vi "大富翁.vi"() -> ()   [LabVIEW 2014]
panel:
  out "白色恐怖?":bool
  out "換誰?":dbl=1.0
  out "按鈕?":dbl
  in  "離開遊戲":bool
  out "骰子":dbl=6.0
  in  "遊戲人數":dbl=4.0
  out "位置 4":dbl
  out "剩幾天 4":dbl
  in  "入獄 4":bool=TRUE
  in  "擲骰子 4":bool
  out "位置 3":dbl
  out "剩幾天 3":dbl
  in  "入獄 3":bool=TRUE
  in  "擲骰子 3":bool
  out "位置 2":dbl
  out "剩幾天 2":dbl
  in  "入獄 2":bool=TRUE
  in  "擲骰子 2":bool
  out "P2指示":bool=TRUE
  out "玩家二財產":dbl
  out "位置 1":dbl
  in  "入獄 1":bool=TRUE
  out "剩幾天 1":dbl
  in  "擲骰子 1":bool=TRUE
  out "P4 棋子":bool=TRUE
  out "P3 棋子":bool=TRUE
  out "P2 棋子":bool=TRUE
  out "P1 棋子":bool
  out "P4指示":bool=TRUE
  out "玩家四財產":dbl
  out "P3指示":bool=TRUE
  out "玩家三財產":dbl
  out "P1指示":bool
  out "玩家一財產":dbl
  in  "中壢市":bool
  in  "新竹市":bool
  in  "新竹縣":bool
  in  "苗栗縣":bool
  in  "台中市":bool
  in  "南投縣":bool
  in  "彰化縣":bool
  in  "雲林縣":bool
  in  "嘉義市":bool
  in  "澎湖縣":bool
  in  "嘉義縣":bool
  in  "阿里山":bool
  in  "台南市":bool
  in  "高雄市":bool
  out "高雄市所有":u32(colorbox)=16777215
  out "中壢市所有":u32(colorbox)=16777215
  out "新竹市所有":u32(colorbox)=16777215
  out "新竹縣所有":u32(colorbox)=16777215
  out "苗栗縣所有":u32(colorbox)=16777215
  out "台中市所有":u32(colorbox)=16777215
  out "南投縣所有":u32(colorbox)=16777215
  out "彰化縣所有":u32(colorbox)=16777215
  out "雲林縣所有":u32(colorbox)=16777215
  out "嘉義市所有":u32(colorbox)=16777215
  out "澎湖縣所有":u32(colorbox)=16777215
  out "嘉義縣所有":u32(colorbox)=16777215
  out "阿里山所有":u32(colorbox)=16777215
  out "台南市所有":u32(colorbox)=16777215
  in  "屏東縣":bool
  out "屏東縣所有":u32(colorbox)=16777215
  in  "¾Á¤B":bool
  out "墾丁所有":u32(colorbox)=16777215
  in  "小琉球":bool
  in  "馬祖":bool
  in  "金門":bool
  in  "蘭嶼":bool
  in  "綠島":bool
  in  "台東縣":bool
  in  "花蓮縣":bool
  in  "宜蘭縣":bool
  in  "基隆市":bool
  in  "台北市":bool
  in  "新北市":bool
  in  "桃園市":bool
  out "桃園市所有":u32(colorbox)=16777215
  out "17旅4":bool
  out "17旅3":bool
  out "17旅2":bool
  out "17旅1":bool
  out "17房4":bool
  out "17房3":bool
  out "17房2":bool
  out "17房1":bool
  out "17¾Á¤B":u32(colorbox)=16777215
  out "19公園":u32(colorbox)=4417863
  out "32入獄":u32(colorbox)=6710886
  out "13監獄":u32(colorbox)=13553358
  out "28命運":u32(colorbox)=12155079
  out "18旅4":bool
  out "18旅3":bool
  out "18旅2":bool
  out "18旅1":bool
  out "18房4":bool
  out "18房3":bool
  out "18房2":bool
  out "18房1":bool
  out "18屏東縣":u32(colorbox)=16777215
  out "16命運":u32(colorbox)=12155079
  out "15旅4":bool
  out "15旅3":bool
  out "15旅2":bool
  out "15旅1":bool
  out "15房4":bool
  out "15房3":bool
  out "15房2":bool
  out "15房1":bool
  out "15小琉球":u32(colorbox)=16777215
  out "35機會":u32(colorbox)=51382
  out "14旅4":bool
  out "14旅3":bool
  out "14旅2":bool
  out "14旅1":bool
  out "14房4":bool
  out "14房3":bool
  out "14房2":bool
  out "14房1":bool
  out "33旅4":bool
  out "33旅3":bool
  out "33旅2":bool
  out "33旅1":bool
  out "33房4":bool
  out "33房3":bool
  out "33房2":bool
  out "33房1":bool
  out "33苗栗縣":u32(colorbox)=16776096
  out "34旅4":bool
  out "34旅3":bool
  out "34旅2":bool
  out "34旅1":bool
  out "34房4":bool
  out "34房3":bool
  out "34房2":bool
  out "34房1":bool
  out "34新竹縣":u32(colorbox)=4377855
  out "36旅4":bool
  out "36旅3":bool
  out "36旅2":bool
  out "36旅1":bool
  out "36房4":bool
  out "36房3":bool
  out "36房2":bool
  out "36房1":bool
  out "36新竹市":u32(colorbox)=10551209
  out "37旅4":bool
  out "37旅3":bool
  out "37旅2":bool
  out "37旅1":bool
  out "37房4":bool
  out "37房3":bool
  out "37房2":bool
  out "37房1":bool
  out "37中壢市":u32(colorbox)=16740729
  out "0起點":u32(colorbox)=16740906
  out "20旅4":bool
  out "20旅3":bool
  out "20旅2":bool
  out "20旅1":bool
  out "20房4":bool
  out "20房3":bool
  out "20房2":bool
  out "20房1":bool
  out "20高雄市":u32(colorbox)=16777215
  out "21旅4":bool
  out "21旅3":bool
  out "21旅2":bool
  out "21旅1":bool
  out "21房4":bool
  out "21房3":bool
  out "21房2":bool
  out "21房1":bool
  out "21台南市":u32(colorbox)=16777215
  out "12旅4":bool
  out "12旅3":bool
  out "12旅2":bool
  out "12旅1":bool
  out "12房4":bool
  out "12房3":bool
  out "12房2":bool
  out "12房1":bool
  out "12金門":u32(colorbox)=16777215
  out "11旅4":bool
  out "11旅3":bool
  out "11旅2":bool
  out "11旅1":bool
  out "11房4":bool
  out "11房3":bool
  out "11房2":bool
  out "11房1":bool
  out "11蘭嶼":u32(colorbox)=16777215
  out "10旅4":bool
  out "10旅3":bool
  out "10旅2":bool
  out "10旅1":bool
  out "10房4":bool
  out "10房3":bool
  out "10房2":bool
  out "10房1":bool
  out "10綠島":u32(colorbox)=16777215
  out "9旅4":bool
  out "9旅3":bool
  out "9旅2":bool
  out "9旅1":bool
  out "9房4":bool
  out "9房3":bool
  out "9房2":bool
  out "9房1":bool
  out "9台東縣":u32(colorbox)=16777215
  out "7旅4":bool
  out "7旅3":bool
  out "7旅2":bool
  out "7旅1":bool
  out "7房4":bool
  out "7房3":bool
  out "7房2":bool
  out "7房1":bool
  out "7花蓮縣":u32(colorbox)=16777215
  out "8機會":u32(colorbox)=51382
  out "5命運":u32(colorbox)=12155079
  out "6旅4":bool
  out "6旅3":bool
  out "6旅2":bool
  out "6旅1":bool
  out "6房4":bool
  out "6房3":bool
  out "6房2":bool
  out "6房1":bool
  out "6宜蘭縣":u32(colorbox)=16777215
  out "4旅4":bool
  out "4旅3":bool
  out "4旅2":bool
  out "4旅1":bool
  out "4房4":bool
  out "4房3":bool
  out "4房2":bool
  out "4房1":bool
  out "4基隆市":u32(colorbox)=16777215
  out "3旅4":bool
  out "3旅3":bool
  out "3旅2":bool
  out "3旅1":bool
  out "3房4":bool
  out "3房3":bool
  out "3房2":bool
  out "3房1":bool
  out "3台北市":u32(colorbox)=16777215
  out "2旅4":bool
  out "2旅3":bool
  out "2旅2":bool
  out "2旅1":bool
  out "2房4":bool
  out "2房3":bool
  out "2房2":bool
  out "2房1":bool
  out "2新北市":u32(colorbox)=16777215
  out "1旅4":bool
  out "1旅3":bool
  out "1旅2":bool
  out "1旅1":bool
  out "1房4":bool
  out "1房3":bool
  out "1房2":bool
  out "1房1":bool
  out "1桃園市":u32(colorbox)=16777215
  out "24機會":u32(colorbox)=51382
  out "22旅4":bool
  out "22旅3":bool
  out "22旅2":bool
  out "22旅1":bool
  out "22房4":bool
  out "22房3":bool
  out "22房2":bool
  out "22房1":bool
  out "22阿里山":u32(colorbox)=16777215
  out "23旅4":bool
  out "23旅3":bool
  out "23旅2":bool
  out "23旅1":bool
  out "23房4":bool
  out "23房3":bool
  out "23房2":bool
  out "23房1":bool
  out "23嘉義縣":u32(colorbox)=16777215
  out "25旅4":bool
  out "25旅3":bool
  out "25旅2":bool
  out "25旅1":bool
  out "25房4":bool
  out "25房3":bool
  out "25房2":bool
  out "25房1":bool
  out "25澎湖縣":u32(colorbox)=16777215
  out "26旅4":bool
  out "26旅3":bool
  out "26旅2":bool
  out "26旅1":bool
  out "26房4":bool
  out "26房3":bool
  out "26房2":bool
  out "26房1":bool
  out "26嘉義市":u32(colorbox)=16777215
  out "27旅4":bool
  out "27旅3":bool
  out "27旅2":bool
  out "27旅1":bool
  out "27房4":bool
  out "27房3":bool
  out "27房2":bool
  out "27房1":bool
  out "29旅4":bool
  out "29旅3":bool
  out "29旅2":bool
  out "29旅1":bool
  out "29房4":bool
  out "29房3":bool
  out "29房2":bool
  out "29房1":bool
  out "29彰化縣":u32(colorbox)=16777215
  out "30旅4":bool
  out "30旅3":bool
  out "30旅2":bool
  out "30旅1":bool
  out "30房4":bool
  out "30房3":bool
  out "30房2":bool
  out "30房1":bool
  out "31旅4":bool
  out "31旅3":bool
  out "31旅2":bool
  out "31旅1":bool
  out "31房4":bool
  out "31房3":bool
  out "31房2":bool
  out "31房1":bool
  out "31台中市":u32(colorbox)=16777215
  out "新北市所有":u32(colorbox)=16777215
  out "小琉球所有":u32(colorbox)=16777215
  out "馬祖所有":u32(colorbox)=16777215
  out "金門縣所有":u32(colorbox)=16777215
  out "蘭嶼所有":u32(colorbox)=16777215
  out "綠島所有":u32(colorbox)=16777215
  out "台東縣所有":u32(colorbox)=16777215
  out "花蓮縣所有":u32(colorbox)=16777215
  out "宜蘭縣所有":u32(colorbox)=16777215
  out "基隆市所有":u32(colorbox)=16777215
  out "台北市所有":u32(colorbox)=16777215
  out "14馬祖":u32(colorbox)=16777215
  out "30南投縣":u32(colorbox)=16777215
  out "27雲林縣":u32(colorbox)=16777215
  out "背景":u32(colorbox)=11121611
  # "起點"
  # "桃園市"
  # "新北市"
  # "台北市"
  # "基隆市"
  # "命運"
  # "宜蘭縣"
  # "花蓮縣"
  # "機會"
  # "台東縣"
  # "綠島"
  # "蘭嶼"
  # "金門"
  # "$1000"
  # "$1500"
  # "$2000"
  # "$750"
  # "$800"
  # "$700"
  # "$650"
  # "$1100"
  # "$800"
  # "$600"
  # "通過+2000!!"
  # "¤¤\nÃc\n¥«"
  # "馬\n祖"
  # "$1000"
  # "$600"
  # "新\n竹\n市"
  # "¤p\n¯[\n²y"
  # "$1300"
  # "$900"
  # "機\n會"
  # "命\n運"
  # "新\n竹\n縣"
  # "¾Á\n¤B"
  # "$900"
  # "$900"
  # "屏\n東\n縣"
  # "­]\n®ß\n¿¤"
  # "$650"
  # "$800"
  # "$1200"
  # "$700"
  # "$750"
  # "$650"
  # "$850"
  # "$900"
  # "$700"
  # "$800"
  # "$1000"
  # "$1800"
  # "台中市"
  # "彰化縣"
  # "嘉義市"
  # "澎湖縣"
  # "機會"
  # "嘉義縣"
  # "阿里山"
  # "台南市"
  # "高雄市"
  # "公園"
  # "入獄"
  # "監獄"
  # "命運"
  # "南投縣"
  # "雲林縣"
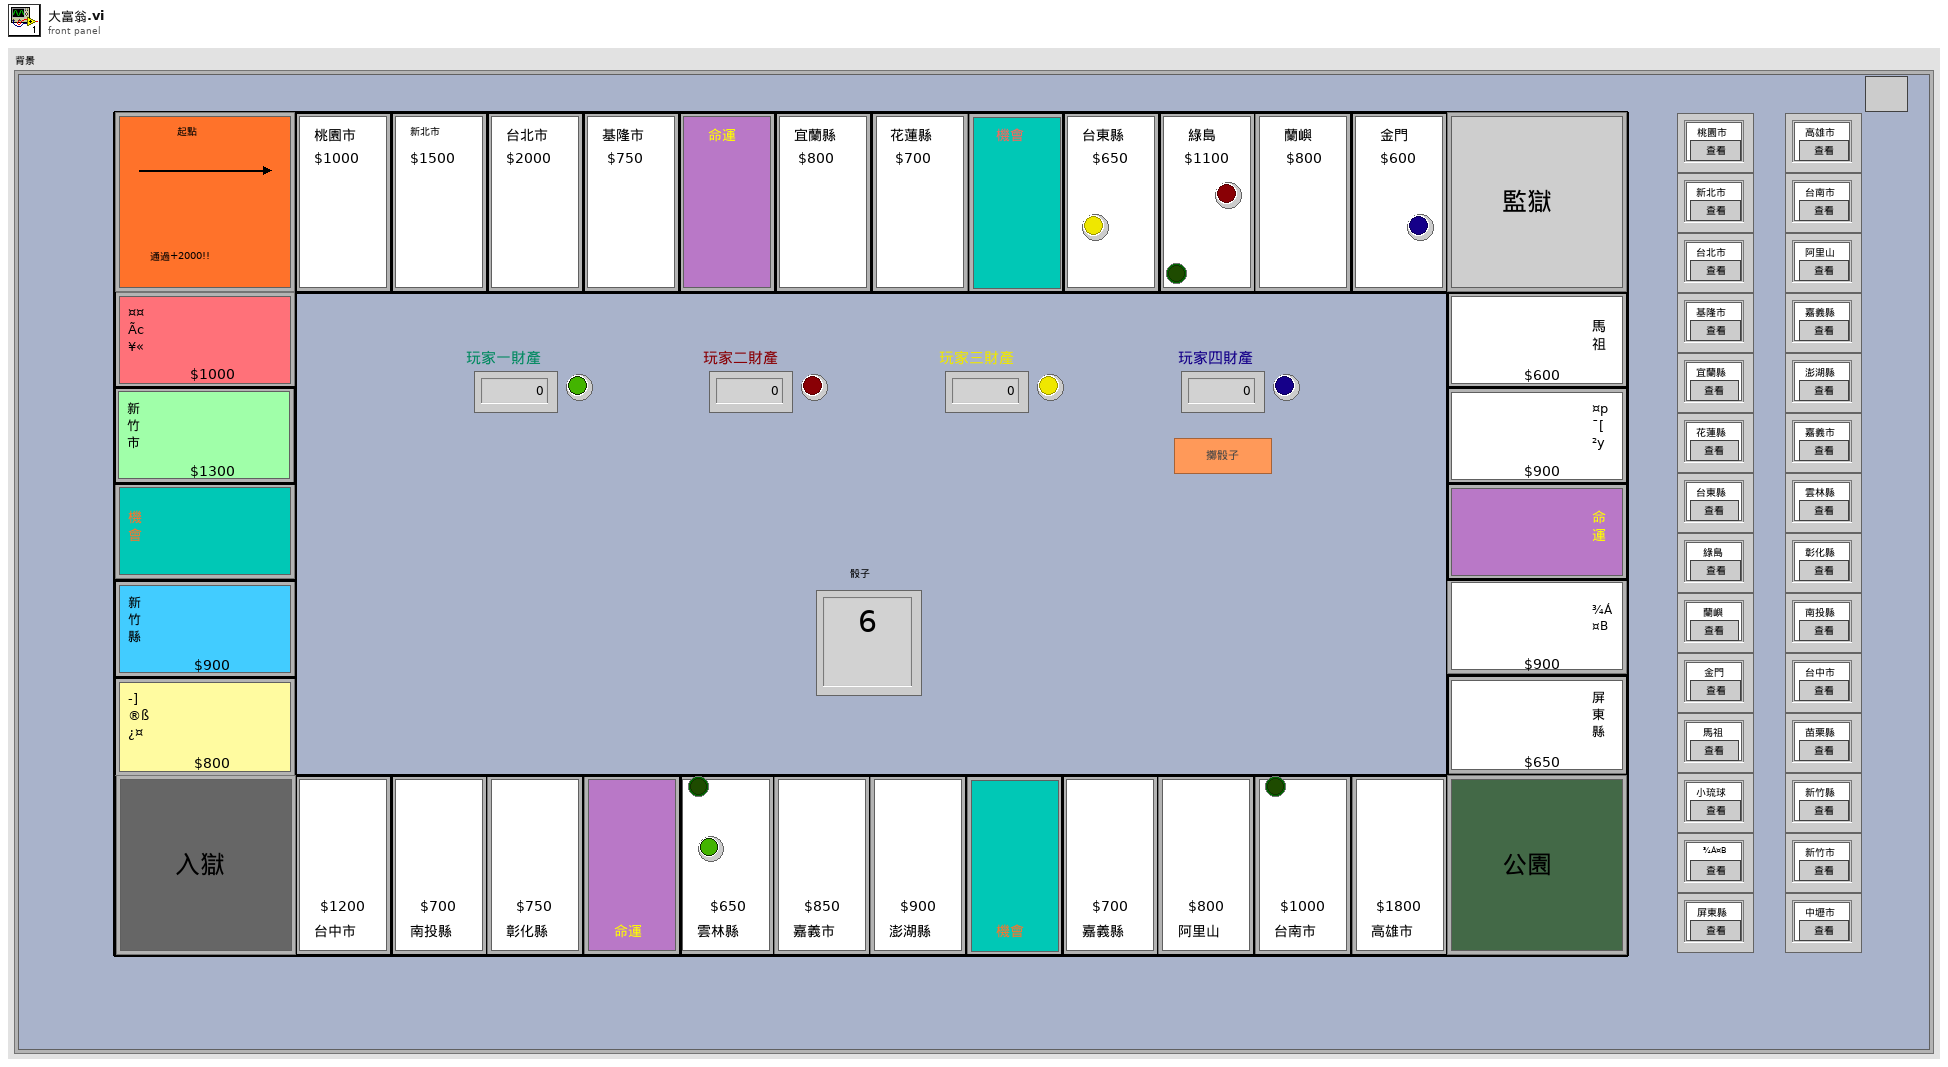
[diagram p1: front panel]
types:
  T1 = enum8{"Enabled", "Disabled", "Disabled and Grayed Out"}
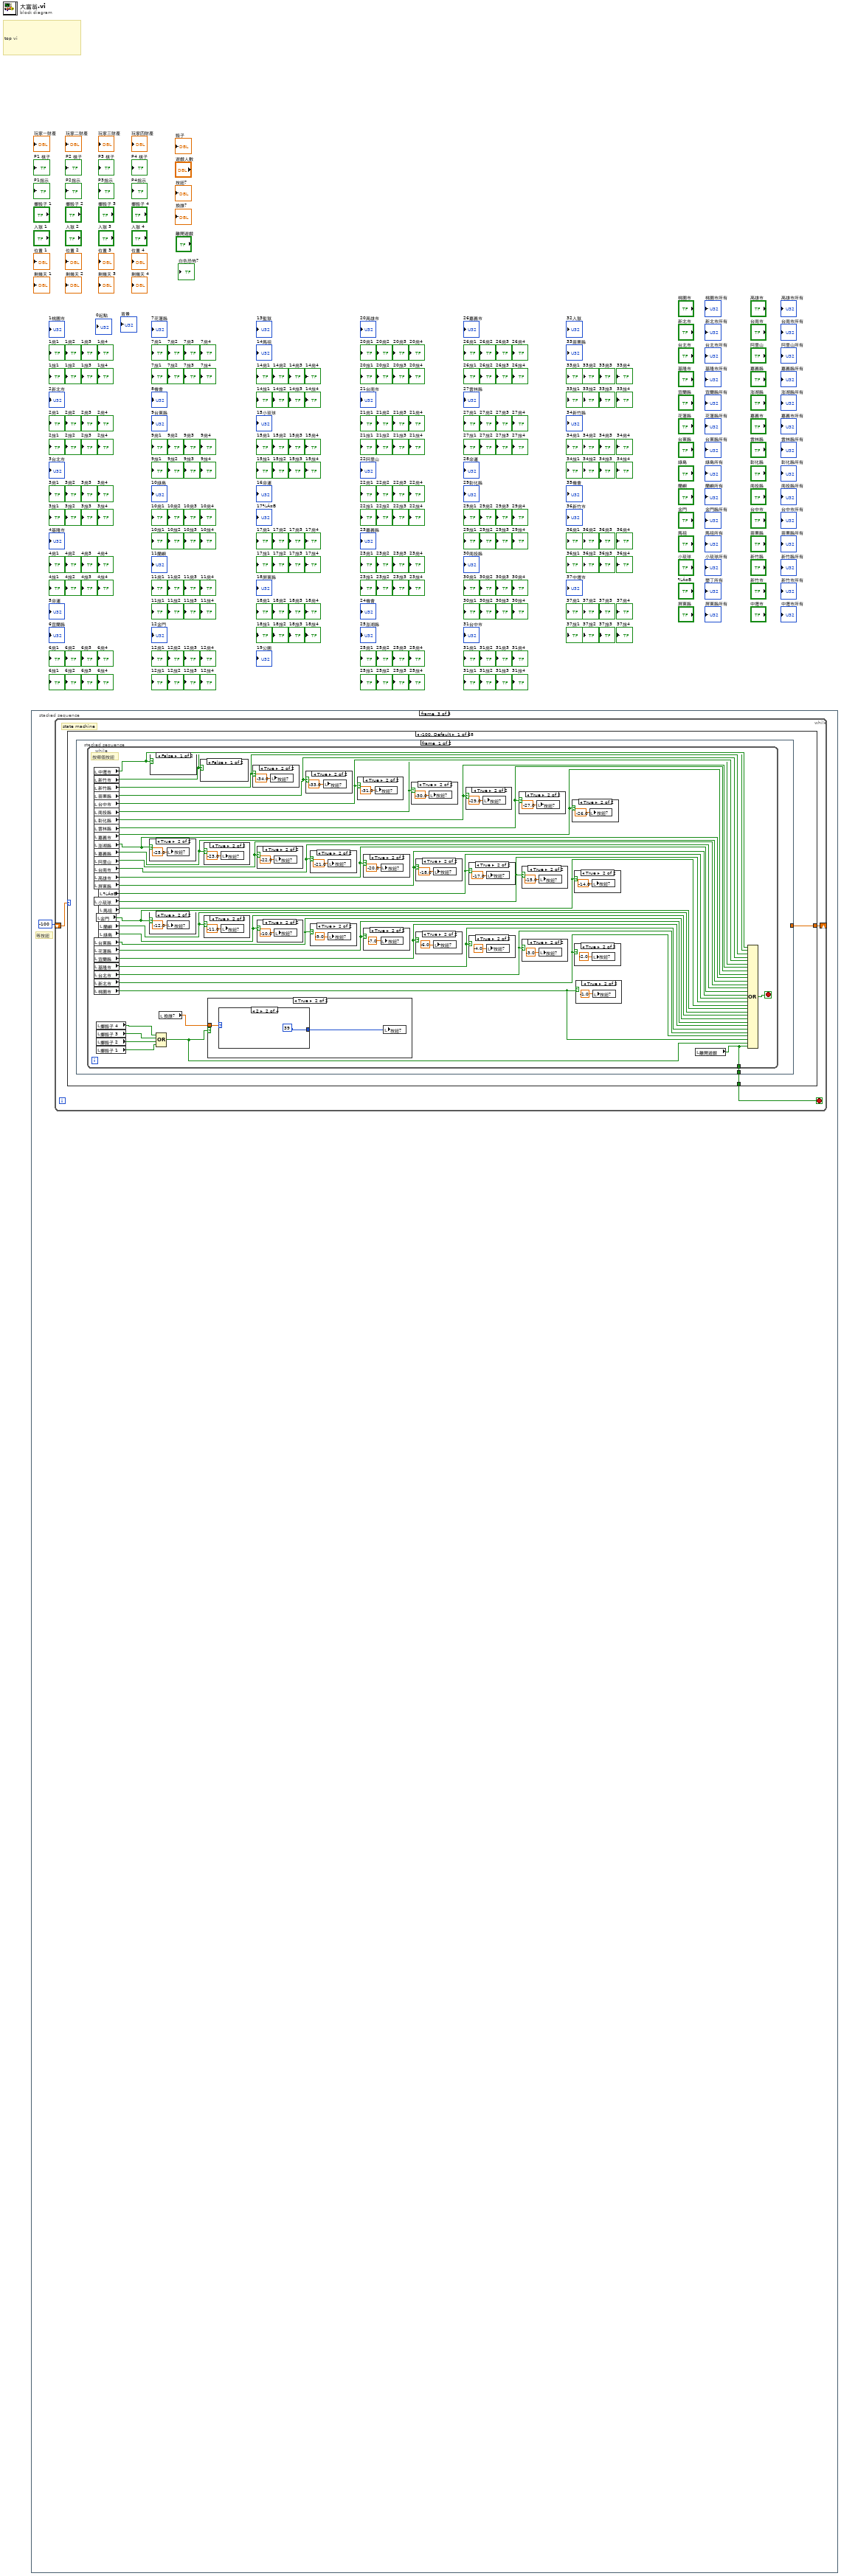
[diagram p0: block diagram]
diagram:
  # "top vi"
  n1 = stacked-sequence {
    frame #0 {
      w3 = TRUE ("P4 棋子")
      w5 = 144 ("Position:Top")
      w6 = 197 ("Position:Left")
      w7 = 112 ("Position:Top")
      w4 = 160 ("Position:Left")
      w8 = 15000.0 ("玩家四財產")
      w9 = FALSE
      w10 = 0.0 ("位置 4")
      w13 = u32 12155079 ("28命運")
      w12 = FALSE ("擲骰子 4")
      w14 = TRUE
      w15 = FALSE
      w17 = FALSE ("Visible")
      w18 = FALSE ("Visible")
      w19 = FALSE ("Visible")
      w20 = FALSE ("Visible")
      w22 = FALSE ("中壢市")
      w21 = FALSE ("Visible")
      w23 = FALSE ("Visible")
      w24 = FALSE
      w25 = u32 16777215 ("中壢市所有")
      w31 = u32 51382 ("地機會")
      w16 = FALSE
      n2 = local write "31旅4"(w16) -> ()
      n3 = local write "31旅3"(w16) -> ()
      n4 = local write "31旅2"(w16) -> ()
      n5 = local write "31旅1"(w16) -> ()
      n6 = local write "31房4"(w16) -> ()
      n7 = local write "31房3"(w16) -> ()
      n8 = local write "31房2"(w16) -> ()
      n9 = local write "31房1"(w16) -> ()
      n10 = local write "30旅4"(w16) -> ()
      n11 = local write "30旅3"(w16) -> ()
      n12 = local write "30旅2"(w16) -> ()
      n13 = local write "30旅1"(w16) -> ()
      n14 = local write "30房4"(w16) -> ()
      n15 = local write "30房3"(w16) -> ()
      n16 = local write "30房2"(w16) -> ()
      n17 = local write "30房1"(w16) -> ()
      n18 = local write "29旅4"(w16) -> ()
      n19 = local write "29旅3"(w16) -> ()
      n20 = local write "29旅2"(w16) -> ()
      n21 = local write "29旅1"(w16) -> ()
      n22 = local write "29房4"(w16) -> ()
      n23 = local write "29房3"(w16) -> ()
      n24 = local write "29房2"(w16) -> ()
      n25 = local write "29房1"(w16) -> ()
      n26 = local write "27旅4"(w16) -> ()
      n27 = local write "27旅3"(w16) -> ()
      n28 = local write "27旅2"(w16) -> ()
      n29 = local write "27旅1"(w16) -> ()
      n30 = local write "27房4"(w16) -> ()
      n31 = local write "27房3"(w16) -> ()
      n32 = local write "27房2"(w16) -> ()
      n33 = local write "27房1"(w16) -> ()
      n34 = local write "26旅4"(w16) -> ()
      n35 = local write "26旅3"(w16) -> ()
      n36 = local write "26旅2"(w16) -> ()
      n37 = local write "26旅1"(w16) -> ()
      n38 = local write "26房4"(w16) -> ()
      n39 = local write "26房3"(w16) -> ()
      n40 = local write "26房2"(w16) -> ()
      n41 = local write "26房1"(w16) -> ()
      n42 = local write "25旅4"(w16) -> ()
      n43 = local write "25旅3"(w16) -> ()
      n44 = local write "25旅2"(w16) -> ()
      n45 = local write "25旅1"(w16) -> ()
      n46 = local write "25房4"(w16) -> ()
      n47 = local write "25房3"(w16) -> ()
      n48 = local write "25房2"(w16) -> ()
      n49 = local write "25房1"(w16) -> ()
      n50 = local write "23旅4"(w16) -> ()
      n51 = local write "23旅3"(w16) -> ()
      n52 = local write "23旅2"(w16) -> ()
      n53 = local write "23旅1"(w16) -> ()
      n54 = local write "23房4"(w16) -> ()
      n55 = local write "23房3"(w16) -> ()
      n56 = local write "23房2"(w16) -> ()
      n57 = local write "23房1"(w16) -> ()
      n58 = local write "22旅4"(w16) -> ()
      n59 = local write "22旅3"(w16) -> ()
      n60 = local write "22旅2"(w16) -> ()
      n61 = local write "22旅1"(w16) -> ()
      n62 = local write "22房4"(w16) -> ()
      n63 = local write "22房3"(w16) -> ()
      n64 = local write "22房2"(w16) -> ()
      n65 = local write "22房1"(w16) -> ()
      n66 = local write "21旅4"(w16) -> ()
      n67 = local write "21旅3"(w16) -> ()
      n68 = local write "21旅2"(w16) -> ()
      n69 = local write "21旅1"(w16) -> ()
      n70 = local write "21房4"(w16) -> ()
      n71 = local write "21房3"(w16) -> ()
      n72 = local write "21房2"(w16) -> ()
      n73 = local write "21房1"(w16) -> ()
      n74 = local write "20旅4"(w16) -> ()
      n75 = local write "20旅3"(w16) -> ()
      n76 = local write "20旅2"(w16) -> ()
      n77 = local write "20旅1"(w16) -> ()
      n78 = local write "20房4"(w16) -> ()
      n79 = local write "20房3"(w16) -> ()
      n80 = local write "20房2"(w16) -> ()
      n81 = local write "20房1"(w16) -> ()
      n82 = local write "1旅4"(w16) -> ()
      n83 = local write "1旅3"(w16) -> ()
      n84 = local write "1旅2"(w16) -> ()
      n85 = local write "1旅1"(w16) -> ()
      n86 = local write "1房4"(w16) -> ()
      n87 = local write "1房3"(w16) -> ()
      n88 = local write "1房2"(w16) -> ()
      n89 = local write "1房1"(w16) -> ()
      n90 = local write "2旅4"(w16) -> ()
      n91 = local write "2旅3"(w16) -> ()
      n92 = local write "2旅2"(w16) -> ()
      n93 = local write "2旅1"(w16) -> ()
      n94 = local write "2房4"(w16) -> ()
      n95 = local write "2房3"(w16) -> ()
      n96 = local write "2房2"(w16) -> ()
      n97 = local write "2房1"(w16) -> ()
      n98 = local write "3旅4"(w16) -> ()
      n99 = local write "3旅3"(w16) -> ()
      n100 = local write "3旅2"(w16) -> ()
      n101 = local write "3旅1"(w16) -> ()
      n102 = local write "3房4"(w16) -> ()
      n103 = local write "3房3"(w16) -> ()
      n104 = local write "3房2"(w16) -> ()
      n105 = local write "3房1"(w16) -> ()
      n106 = local write "4旅4"(w16) -> ()
      n107 = local write "4旅3"(w16) -> ()
      n108 = local write "4旅2"(w16) -> ()
      n109 = local write "4旅1"(w16) -> ()
      n110 = local write "4房4"(w16) -> ()
      n111 = local write "4房3"(w16) -> ()
      n112 = local write "4房2"(w16) -> ()
      n113 = local write "4房1"(w16) -> ()
      n114 = local write "6旅4"(w16) -> ()
      n115 = local write "6旅3"(w16) -> ()
      n116 = local write "6旅2"(w16) -> ()
      n117 = local write "6旅1"(w16) -> ()
      n118 = local write "6房4"(w16) -> ()
      n119 = local write "6房3"(w16) -> ()
      n120 = local write "6房2"(w16) -> ()
      n121 = local write "6房1"(w16) -> ()
      n122 = local write "7旅4"(w16) -> ()
      n123 = local write "7旅3"(w16) -> ()
      n124 = local write "7旅2"(w16) -> ()
      n125 = local write "7旅1"(w16) -> ()
      n126 = local write "7房4"(w16) -> ()
      n127 = local write "7房3"(w16) -> ()
      n128 = local write "7房2"(w16) -> ()
      n129 = local write "7房1"(w16) -> ()
      n130 = local write "9旅4"(w16) -> ()
      n131 = local write "9旅3"(w16) -> ()
      n132 = local write "9旅2"(w16) -> ()
      n133 = local write "9旅1"(w16) -> ()
      n134 = local write "9房4"(w16) -> ()
      n135 = local write "9房3"(w16) -> ()
      n136 = local write "9房2"(w16) -> ()
      n137 = local write "9房1"(w16) -> ()
      n138 = local write "10旅4"(w16) -> ()
      n139 = local write "10旅3"(w16) -> ()
      n140 = local write "10旅2"(w16) -> ()
      n141 = local write "10旅1"(w16) -> ()
      n142 = local write "10房4"(w16) -> ()
      n143 = local write "10房3"(w16) -> ()
      n144 = local write "10房2"(w16) -> ()
      n145 = local write "10房1"(w16) -> ()
      n146 = local write "11旅4"(w16) -> ()
      n147 = local write "11旅3"(w16) -> ()
      n148 = local write "11旅2"(w16) -> ()
      n149 = local write "11旅1"(w16) -> ()
      n150 = local write "11房4"(w16) -> ()
      n151 = local write "11房3"(w16) -> ()
      n152 = local write "11房2"(w16) -> ()
      n153 = local write "11房1"(w16) -> ()
      n154 = local write "12旅4"(w16) -> ()
      n155 = local write "12旅3"(w16) -> ()
      n156 = local write "12旅2"(w16) -> ()
      n157 = local write "12旅1"(w16) -> ()
      n158 = local write "12房4"(w16) -> ()
      n159 = local write "12房3"(w16) -> ()
      n160 = local write "12房2"(w16) -> ()
      n161 = local write "12房1"(w16) -> ()
      n162 = local write "37旅4"(w16) -> ()
      n163 = local write "37旅3"(w16) -> ()
      n164 = local write "37旅2"(w16) -> ()
      n165 = local write "37旅1"(w16) -> ()
      n166 = local write "37房4"(w16) -> ()
      n167 = local write "37房3"(w16) -> ()
      n168 = local write "37房2"(w16) -> ()
      n169 = local write "37房1"(w16) -> ()
      n170 = local write "36旅4"(w16) -> ()
      n171 = local write "36旅3"(w16) -> ()
      n172 = local write "36旅2"(w16) -> ()
      n173 = local write "36旅1"(w16) -> ()
      n174 = local write "36房4"(w16) -> ()
      n175 = local write "36房3"(w16) -> ()
      n176 = local write "36房2"(w16) -> ()
      n177 = local write "36房1"(w16) -> ()
      n178 = local write "34旅4"(w16) -> ()
      n179 = local write "34旅3"(w16) -> ()
      n180 = local write "34旅2"(w16) -> ()
      n181 = local write "34旅1"(w16) -> ()
      n182 = local write "34房4"(w16) -> ()
      n183 = local write "34房3"(w16) -> ()
      n184 = local write "34房2"(w16) -> ()
      n185 = local write "34房1"(w16) -> ()
      n186 = local write "33旅4"(w16) -> ()
      n187 = local write "33旅3"(w16) -> ()
      n188 = local write "33旅2"(w16) -> ()
      n189 = local write "33旅1"(w16) -> ()
      n190 = local write "33房4"(w16) -> ()
      n191 = local write "33房3"(w16) -> ()
      n192 = local write "33房2"(w16) -> ()
      n193 = local write "33房1"(w16) -> ()
      n194 = local write "18旅4"(w16) -> ()
      n195 = local write "18旅3"(w16) -> ()
      n196 = local write "18旅2"(w16) -> ()
      n197 = local write "18旅1"(w16) -> ()
      n198 = local write "18房4"(w16) -> ()
      n199 = local write "18房3"(w16) -> ()
      n200 = local write "18房2"(w16) -> ()
      n201 = local write "18房1"(w16) -> ()
      n202 = local write "17旅4"(w16) -> ()
      n203 = local write "17旅3"(w16) -> ()
      n204 = local write "17旅2"(w16) -> ()
      n205 = local write "17旅1"(w16) -> ()
      n206 = local write "17房4"(w16) -> ()
      n207 = local write "17房3"(w16) -> ()
      n208 = local write "17房2"(w16) -> ()
      n209 = local write "17房1"(w16) -> ()
      n210 = local write "15旅4"(w16) -> ()
      n211 = local write "15旅3"(w16) -> ()
      n212 = local write "15旅2"(w16) -> ()
      n213 = local write "15旅1"(w16) -> ()
      n214 = local write "15房4"(w16) -> ()
      n215 = local write "15房3"(w16) -> ()
      n216 = local write "15房2"(w16) -> ()
      n217 = local write "15房1"(w16) -> ()
      n218 = local write "14旅4"(w16) -> ()
      n219 = local write "14旅3"(w16) -> ()
      n220 = local write "14旅2"(w16) -> ()
      n221 = local write "14旅1"(w16) -> ()
      n222 = local write "14房4"(w16) -> ()
      n223 = local write "14房3"(w16) -> ()
      n224 = local write "14房2"(w16) -> ()
      n225 = local write "14房1"(w16) -> ()
      n226 = local write "19公園"(u32 4417863 ("公園")) -> ()
      n227 = local write "32入獄"(u32 6710886 ("入獄")) -> ()
      n228 = local write "13監獄"(u32 13553358 ("監獄")) -> ()
      n229 = local write "0起點"(u32 16740906 ("起點")) -> ()
      n230 = local write "中壢市所有"(w25) -> ()
      n231 = local write "新竹市所有"(w25) -> ()
      n232 = local write "新竹縣所有"(w25) -> ()
      n233 = local write "苗栗縣所有"(w25) -> ()
      n234 = local write "台中市所有"(w25) -> ()
      n235 = local write "南投縣所有"(w25) -> ()
      n236 = local write "彰化縣所有"(w25) -> ()
      n237 = local write "雲林縣所有"(w25) -> ()
      n238 = local write "嘉義市所有"(w25) -> ()
      n239 = local write "澎湖縣所有"(w25) -> ()
      n240 = local write "嘉義縣所有"(w25) -> ()
      n241 = local write "阿里山所有"(w25) -> ()
      n242 = local write "台南市所有"(w25) -> ()
      n243 = local write "高雄市所有"(w25) -> ()
      n244 = local write "屏東縣所有"(w25) -> ()
      n245 = local write "墾丁所有"(w25) -> ()
      n246 = local write "小琉球所有"(w25) -> ()
      n247 = local write "馬祖所有"(w25) -> ()
      n248 = local write "金門縣所有"(w25) -> ()
      n249 = local write "蘭嶼所有"(w25) -> ()
      n250 = local write "綠島所有"(w25) -> ()
      n251 = local write "台東縣所有"(w25) -> ()
      n252 = local write "花蓮縣所有"(w25) -> ()
      n253 = local write "宜蘭縣所有"(w25) -> ()
      n254 = local write "基隆市所有"(w25) -> ()
      n255 = local write "台北市所有"(w25) -> ()
      n256 = local write "新北市所有"(w25) -> ()
      n257 = local write "桃園市所有"(w25) -> ()
      n258 = local write "31台中市"(w25) -> ()
      n259 = local write "25澎湖縣"(w25) -> ()
      n260 = local write "30南投縣"(w25) -> ()
      n261 = local write "29彰化縣"(w25) -> ()
      n262 = local write "27雲林縣"(w25) -> ()
      n263 = local write "26嘉義市"(w25) -> ()
      n264 = local write "23嘉義縣"(w25) -> ()
      n265 = local write "22阿里山"(w25) -> ()
      n266 = local write "21台南市"(w25) -> ()
      n267 = local write "20高雄市"(w25) -> ()
      n268 = local write "1桃園市"(w25) -> ()
      n269 = local write "2新北市"(w25) -> ()
      n270 = local write "3台北市"(w25) -> ()
      n271 = local write "4基隆市"(w25) -> ()
      n272 = local write "6宜蘭縣"(w25) -> ()
      n273 = local write "12金門"(w25) -> ()
      n274 = local write "11蘭嶼"(w25) -> ()
      n275 = local write "10綠島"(w25) -> ()
      n276 = local write "9台東縣"(w25) -> ()
      n277 = local write "7花蓮縣"(w25) -> ()
      n278 = local write "37中壢市"(w25) -> ()
      n279 = local write "36新竹市"(w25) -> ()
      n280 = local write "34新竹縣"(w25) -> ()
      n281 = local write "33苗栗縣"(w25) -> ()
      n282 = local write "14馬祖"(w25) -> ()
      n283 = local write "15小琉球"(w25) -> ()
      n284 = local write "17¾Á¤B"(w25) -> ()
      n285 = local write "18屏東縣"(w25) -> ()
      n286 = local write "28命運"(w13) -> ()
      n287 = local write "5命運"(w13) -> ()
      n288 = local write "16命運"(w13) -> ()
      n289 = local write "35機會"(w31) -> ()
      n290 = local write "8機會"(w31) -> ()
      n291 = local write "24機會"(w31) -> ()
      n292 = local write "P4 棋子"(w3) -> ()
      n293 = local write "P3 棋子"(w3) -> ()
      n294 = local write "P2 棋子"(w3) -> ()
      n295 = local write "P1 棋子"(w3) -> ()
      n296 = local write "P1指示"(w3) -> ()
      n297 = local write "P2指示"(w3) -> ()
      n298 = local write "P3指示"(w3) -> ()
      n299 = local write "P4指示"(w3) -> ()
      n300 = local write "背景"(u32 11121611 ("背景")) -> ()
      n301 = property on="背景" class="ColBox"("Visible"=w3) -> ()  [unwired: 2 in, 2 out]
      n302 = Increment(x=w10) -> (x+1=w11:dbl)
      n303 = local write "中壢市"(w22) -> ()
      n304 = local write "新竹市"(w22) -> ()
      n305 = local write "新竹縣"(w22) -> ()
      n306 = local write "苗栗縣"(w22) -> ()
      n307 = local write "台中市"(w22) -> ()
      n308 = local write "南投縣"(w22) -> ()
      n309 = local write "彰化縣"(w22) -> ()
      n310 = local write "雲林縣"(w22) -> ()
      n311 = local write "嘉義市"(w22) -> ()
      n312 = local write "澎湖縣"(w22) -> ()
      n313 = local write "嘉義縣"(w22) -> ()
      n314 = local write "阿里山"(w22) -> ()
      n315 = local write "台南市"(w22) -> ()
      n316 = local write "高雄市"(w22) -> ()
      n317 = local write "屏東縣"(w22) -> ()
      n318 = local write "¾Á¤B"(w22) -> ()
      n319 = local write "小琉球"(w22) -> ()
      n320 = local write "馬祖"(w22) -> ()
      n321 = local write "金門"(w22) -> ()
      n322 = local write "蘭嶼"(w22) -> ()
      n323 = local write "綠島"(w22) -> ()
      n324 = local write "台東縣"(w22) -> ()
      n325 = local write "花蓮縣"(w22) -> ()
      n326 = local write "宜蘭縣"(w22) -> ()
      n327 = local write "基隆市"(w22) -> ()
      n328 = local write "台北市"(w22) -> ()
      n329 = local write "新北市"(w22) -> ()
      n330 = local write "桃園市"(w22) -> ()
      n331 = local write "位置 4"(w10) -> ()
      n332 = local write "剩幾天 4"(w10) -> ()
      n333 = local write "位置 3"(w10) -> ()
      n334 = local write "剩幾天 3"(w10) -> ()
      n335 = local write "位置 2"(w10) -> ()
      n336 = local write "剩幾天 2"(w10) -> ()
      n337 = local write "位置 1"(w10) -> ()
      n338 = local write "剩幾天 1"(w10) -> ()
      n339 = local write "按鈕?"(w10) -> ()
      n340 = local write "換誰?"(w11) -> ()
      n341 = local write "玩家四財產"(w8) -> ()
      n342 = local write "玩家三財產"(w8) -> ()
      n343 = local write "玩家二財產"(w8) -> ()
      n344 = local write "玩家一財產"(w8) -> ()
      n345 = property on="P1 棋子" class="Bool (strict)"("Left"=w4, "Top"=w7) -> ()  [unwired: 2 in, 2 out]
      n346 = property on="P2 棋子" class="Bool (strict)"("Left"=w6, "Top"=w7) -> ()  [unwired: 2 in, 2 out]
      n347 = property on="P3 棋子" class="Bool (strict)"("Left"=w4, "Top"=w5) -> ()  [unwired: 2 in, 2 out]
      n348 = property on="P4 棋子" class="Bool (strict)"("Left"=w6, "Top"=w5) -> ()  [unwired: 2 in, 2 out]
      n349 = property on="1房1" class="Bool (strict)"("Visible"=w24) -> ()  [unwired: 2 in, 2 out]
      n350 = property on="1房2" class="Bool (strict)"("Visible"=w24) -> ()  [unwired: 2 in, 2 out]
      n351 = property on="1房3" class="Bool (strict)"("Visible"=w24) -> ()  [unwired: 2 in, 2 out]
      n352 = property on="1房4" class="Bool (strict)"("Visible"=w24) -> ()  [unwired: 2 in, 2 out]
      n353 = property on="1旅1" class="Bool (strict)"("Visible"=w24) -> ()  [unwired: 2 in, 2 out]
      n354 = property on="1旅2" class="Bool (strict)"("Visible"=w24) -> ()  [unwired: 2 in, 2 out]
      n355 = property on="1旅3" class="Bool (strict)"("Visible"=w24) -> ()  [unwired: 2 in, 2 out]
      n356 = property on="1旅4" class="Bool (strict)"("Visible"=w24) -> ()  [unwired: 2 in, 2 out]
      n357 = property on="2房1" class="Bool (strict)"("Visible"=w24) -> ()  [unwired: 2 in, 2 out]
      n358 = property on="2房2" class="Bool (strict)"("Visible"=w24) -> ()  [unwired: 2 in, 2 out]
      n359 = property on="2房3" class="Bool (strict)"("Visible"=w24) -> ()  [unwired: 2 in, 2 out]
      n360 = property on="2房4" class="Bool (strict)"("Visible"=w24) -> ()  [unwired: 2 in, 2 out]
      n361 = property on="2旅1" class="Bool (strict)"("Visible"=w24) -> ()  [unwired: 2 in, 2 out]
      n362 = property on="2旅2" class="Bool (strict)"("Visible"=w24) -> ()  [unwired: 2 in, 2 out]
      n363 = property on="2旅3" class="Bool (strict)"("Visible"=w24) -> ()  [unwired: 2 in, 2 out]
      n364 = property on="2旅4" class="Bool (strict)"("Visible"=w24) -> ()  [unwired: 2 in, 2 out]
      n365 = property on="3房1" class="Bool (strict)"("Visible"=w24) -> ()  [unwired: 2 in, 2 out]
      n366 = property on="3房2" class="Bool (strict)"("Visible"=w24) -> ()  [unwired: 2 in, 2 out]
      n367 = property on="3房3" class="Bool (strict)"("Visible"=w24) -> ()  [unwired: 2 in, 2 out]
      n368 = property on="3房4" class="Bool (strict)"("Visible"=w24) -> ()  [unwired: 2 in, 2 out]
      n369 = property on="3旅1" class="Bool (strict)"("Visible"=w24) -> ()  [unwired: 2 in, 2 out]
      n370 = property on="3旅2" class="Bool (strict)"("Visible"=w24) -> ()  [unwired: 2 in, 2 out]
      n371 = property on="3旅3" class="Bool (strict)"("Visible"=w24) -> ()  [unwired: 2 in, 2 out]
      n372 = property on="3旅4" class="Bool (strict)"("Visible"=w24) -> ()  [unwired: 2 in, 2 out]
      n373 = property on="4房1" class="Bool (strict)"("Visible"=w24) -> ()  [unwired: 2 in, 2 out]
      n374 = property on="4房2" class="Bool (strict)"("Visible"=w24) -> ()  [unwired: 2 in, 2 out]
      n375 = property on="4房3" class="Bool (strict)"("Visible"=w24) -> ()  [unwired: 2 in, 2 out]
      n376 = property on="4房4" class="Bool (strict)"("Visible"=w24) -> ()  [unwired: 2 in, 2 out]
      n377 = property on="4旅1" class="Bool (strict)"("Visible"=w24) -> ()  [unwired: 2 in, 2 out]
      n378 = property on="4旅2" class="Bool (strict)"("Visible"=w24) -> ()  [unwired: 2 in, 2 out]
      n379 = property on="4旅3" class="Bool (strict)"("Visible"=w24) -> ()  [unwired: 2 in, 2 out]
      n380 = property on="4旅4" class="Bool (strict)"("Visible"=w24) -> ()  [unwired: 2 in, 2 out]
      n381 = property on="6房1" class="Bool (strict)"("Visible"=w23) -> ()  [unwired: 2 in, 2 out]
      n382 = property on="6房2" class="Bool (strict)"("Visible"=w23) -> ()  [unwired: 2 in, 2 out]
      n383 = property on="6房3" class="Bool (strict)"("Visible"=w23) -> ()  [unwired: 2 in, 2 out]
      n384 = property on="6房4" class="Bool (strict)"("Visible"=w23) -> ()  [unwired: 2 in, 2 out]
      n385 = property on="6旅1" class="Bool (strict)"("Visible"=w23) -> ()  [unwired: 2 in, 2 out]
      n386 = property on="6旅2" class="Bool (strict)"("Visible"=w23) -> ()  [unwired: 2 in, 2 out]
      n387 = property on="6旅3" class="Bool (strict)"("Visible"=w23) -> ()  [unwired: 2 in, 2 out]
      n388 = property on="6旅4" class="Bool (strict)"("Visible"=w23) -> ()  [unwired: 2 in, 2 out]
      n389 = property on="7房1" class="Bool (strict)"("Visible"=w23) -> ()  [unwired: 2 in, 2 out]
      n390 = property on="7房2" class="Bool (strict)"("Visible"=w23) -> ()  [unwired: 2 in, 2 out]
      n391 = property on="7房3" class="Bool (strict)"("Visible"=w23) -> ()  [unwired: 2 in, 2 out]
      n392 = property on="7房4" class="Bool (strict)"("Visible"=w23) -> ()  [unwired: 2 in, 2 out]
      n393 = property on="7旅1" class="Bool (strict)"("Visible"=w23) -> ()  [unwired: 2 in, 2 out]
      n394 = property on="7旅2" class="Bool (strict)"("Visible"=w23) -> ()  [unwired: 2 in, 2 out]
      n395 = property on="7旅3" class="Bool (strict)"("Visible"=w23) -> ()  [unwired: 2 in, 2 out]
      n396 = property on="7旅4" class="Bool (strict)"("Visible"=w23) -> ()  [unwired: 2 in, 2 out]
      n397 = property on="9房1" class="Bool (strict)"("Visible"=w23) -> ()  [unwired: 2 in, 2 out]
      n398 = property on="9房2" class="Bool (strict)"("Visible"=w23) -> ()  [unwired: 2 in, 2 out]
      n399 = property on="9房3" class="Bool (strict)"("Visible"=w23) -> ()  [unwired: 2 in, 2 out]
      n400 = property on="9房4" class="Bool (strict)"("Visible"=w23) -> ()  [unwired: 2 in, 2 out]
      n401 = property on="9旅1" class="Bool (strict)"("Visible"=w23) -> ()  [unwired: 2 in, 2 out]
      n402 = property on="9旅2" class="Bool (strict)"("Visible"=w23) -> ()  [unwired: 2 in, 2 out]
      n403 = property on="9旅3" class="Bool (strict)"("Visible"=w23) -> ()  [unwired: 2 in, 2 out]
      n404 = property on="9旅4" class="Bool (strict)"("Visible"=w23) -> ()  [unwired: 2 in, 2 out]
      n405 = property on="10房1" class="Bool (strict)"("Visible"=w23) -> ()  [unwired: 2 in, 2 out]
      n406 = property on="10房2" class="Bool (strict)"("Visible"=w23) -> ()  [unwired: 2 in, 2 out]
      n407 = property on="10房3" class="Bool (strict)"("Visible"=w23) -> ()  [unwired: 2 in, 2 out]
      n408 = property on="10房4" class="Bool (strict)"("Visible"=w23) -> ()  [unwired: 2 in, 2 out]
      n409 = property on="10旅1" class="Bool (strict)"("Visible"=w23) -> ()  [unwired: 2 in, 2 out]
      n410 = property on="10旅2" class="Bool (strict)"("Visible"=w23) -> ()  [unwired: 2 in, 2 out]
      n411 = property on="10旅3" class="Bool (strict)"("Visible"=w23) -> ()  [unwired: 2 in, 2 out]
      n412 = property on="10旅4" class="Bool (strict)"("Visible"=w23) -> ()  [unwired: 2 in, 2 out]
      n413 = property on="11房1" class="Bool (strict)"("Visible"=w21) -> ()  [unwired: 2 in, 2 out]
      n414 = property on="11房2" class="Bool (strict)"("Visible"=w21) -> ()  [unwired: 2 in, 2 out]
      n415 = property on="11房3" class="Bool (strict)"("Visible"=w21) -> ()  [unwired: 2 in, 2 out]
      n416 = property on="11房4" class="Bool (strict)"("Visible"=w21) -> ()  [unwired: 2 in, 2 out]
      n417 = property on="11旅1" class="Bool (strict)"("Visible"=w21) -> ()  [unwired: 2 in, 2 out]
      n418 = property on="11旅2" class="Bool (strict)"("Visible"=w21) -> ()  [unwired: 2 in, 2 out]
      n419 = property on="11旅3" class="Bool (strict)"("Visible"=w21) -> ()  [unwired: 2 in, 2 out]
      n420 = property on="11旅4" class="Bool (strict)"("Visible"=w21) -> ()  [unwired: 2 in, 2 out]
      n421 = property on="12房1" class="Bool (strict)"("Visible"=w21) -> ()  [unwired: 2 in, 2 out]
      n422 = property on="12房2" class="Bool (strict)"("Visible"=w21) -> ()  [unwired: 2 in, 2 out]
      n423 = property on="12房3" class="Bool (strict)"("Visible"=w21) -> ()  [unwired: 2 in, 2 out]
      n424 = property on="12房4" class="Bool (strict)"("Visible"=w21) -> ()  [unwired: 2 in, 2 out]
      n425 = property on="12旅1" class="Bool (strict)"("Visible"=w21) -> ()  [unwired: 2 in, 2 out]
      n426 = property on="12旅2" class="Bool (strict)"("Visible"=w21) -> ()  [unwired: 2 in, 2 out]
      n427 = property on="12旅3" class="Bool (strict)"("Visible"=w21) -> ()  [unwired: 2 in, 2 out]
      n428 = property on="12旅4" class="Bool (strict)"("Visible"=w21) -> ()  [unwired: 2 in, 2 out]
      n429 = property on="14房1" class="Bool (strict)"("Visible"=w21) -> ()  [unwired: 2 in, 2 out]
      n430 = property on="14房2" class="Bool (strict)"("Visible"=w21) -> ()  [unwired: 2 in, 2 out]
      n431 = property on="14房3" class="Bool (strict)"("Visible"=w21) -> ()  [unwired: 2 in, 2 out]
      n432 = property on="14房4" class="Bool (strict)"("Visible"=w21) -> ()  [unwired: 2 in, 2 out]
      n433 = property on="14旅1" class="Bool (strict)"("Visible"=w21) -> ()  [unwired: 2 in, 2 out]
      n434 = property on="14旅2" class="Bool (strict)"("Visible"=w21) -> ()  [unwired: 2 in, 2 out]
      n435 = property on="14旅3" class="Bool (strict)"("Visible"=w21) -> ()  [unwired: 2 in, 2 out]
      n436 = property on="14旅4" class="Bool (strict)"("Visible"=w21) -> ()  [unwired: 2 in, 2 out]
      n437 = property on="15房1" class="Bool (strict)"("Visible"=w21) -> ()  [unwired: 2 in, 2 out]
      n438 = property on="15房2" class="Bool (strict)"("Visible"=w21) -> ()  [unwired: 2 in, 2 out]
      n439 = property on="15房3" class="Bool (strict)"("Visible"=w21) -> ()  [unwired: 2 in, 2 out]
      n440 = property on="15房4" class="Bool (strict)"("Visible"=w21) -> ()  [unwired: 2 in, 2 out]
      n441 = property on="15旅1" class="Bool (strict)"("Visible"=w21) -> ()  [unwired: 2 in, 2 out]
      n442 = property on="15旅2" class="Bool (strict)"("Visible"=w21) -> ()  [unwired: 2 in, 2 out]
      n443 = property on="15旅3" class="Bool (strict)"("Visible"=w21) -> ()  [unwired: 2 in, 2 out]
      n444 = property on="15旅4" class="Bool (strict)"("Visible"=w21) -> ()  [unwired: 2 in, 2 out]
      n445 = property on="17房1" class="Bool (strict)"("Visible"=w20) -> ()  [unwired: 2 in, 2 out]
      n446 = property on="17房2" class="Bool (strict)"("Visible"=w20) -> ()  [unwired: 2 in, 2 out]
      n447 = property on="17房3" class="Bool (strict)"("Visible"=w20) -> ()  [unwired: 2 in, 2 out]
      n448 = property on="17房4" class="Bool (strict)"("Visible"=w20) -> ()  [unwired: 2 in, 2 out]
      n449 = property on="17旅1" class="Bool (strict)"("Visible"=w20) -> ()  [unwired: 2 in, 2 out]
      n450 = property on="17旅2" class="Bool (strict)"("Visible"=w20) -> ()  [unwired: 2 in, 2 out]
      n451 = property on="17旅3" class="Bool (strict)"("Visible"=w20) -> ()  [unwired: 2 in, 2 out]
      n452 = property on="17旅4" class="Bool (strict)"("Visible"=w20) -> ()  [unwired: 2 in, 2 out]
      n453 = property on="18房1" class="Bool (strict)"("Visible"=w20) -> ()  [unwired: 2 in, 2 out]
      n454 = property on="18房2" class="Bool (strict)"("Visible"=w20) -> ()  [unwired: 2 in, 2 out]
      n455 = property on="18房3" class="Bool (strict)"("Visible"=w20) -> ()  [unwired: 2 in, 2 out]
      n456 = property on="18房4" class="Bool (strict)"("Visible"=w20) -> ()  [unwired: 2 in, 2 out]
      n457 = property on="18旅1" class="Bool (strict)"("Visible"=w20) -> ()  [unwired: 2 in, 2 out]
      n458 = property on="18旅2" class="Bool (strict)"("Visible"=w20) -> ()  [unwired: 2 in, 2 out]
      n459 = property on="18旅3" class="Bool (strict)"("Visible"=w20) -> ()  [unwired: 2 in, 2 out]
      n460 = property on="18旅4" class="Bool (strict)"("Visible"=w20) -> ()  [unwired: 2 in, 2 out]
      n461 = property on="20房1" class="Bool (strict)"("Visible"=w20) -> ()  [unwired: 2 in, 2 out]
      n462 = property on="20房2" class="Bool (strict)"("Visible"=w20) -> ()  [unwired: 2 in, 2 out]
      n463 = property on="20房3" class="Bool (strict)"("Visible"=w20) -> ()  [unwired: 2 in, 2 out]
      n464 = property on="20房4" class="Bool (strict)"("Visible"=w20) -> ()  [unwired: 2 in, 2 out]
      n465 = property on="20旅1" class="Bool (strict)"("Visible"=w20) -> ()  [unwired: 2 in, 2 out]
      n466 = property on="20旅2" class="Bool (strict)"("Visible"=w20) -> ()  [unwired: 2 in, 2 out]
      n467 = property on="20旅3" class="Bool (strict)"("Visible"=w20) -> ()  [unwired: 2 in, 2 out]
      n468 = property on="20旅4" class="Bool (strict)"("Visible"=w20) -> ()  [unwired: 2 in, 2 out]
      n469 = property on="21房1" class="Bool (strict)"("Visible"=w20) -> ()  [unwired: 2 in, 2 out]
      n470 = property on="21房2" class="Bool (strict)"("Visible"=w20) -> ()  [unwired: 2 in, 2 out]
      n471 = property on="21房3" class="Bool (strict)"("Visible"=w20) -> ()  [unwired: 2 in, 2 out]
      n472 = property on="21房4" class="Bool (strict)"("Visible"=w20) -> ()  [unwired: 2 in, 2 out]
      n473 = property on="21旅1" class="Bool (strict)"("Visible"=w20) -> ()  [unwired: 2 in, 2 out]
      n474 = property on="21旅2" class="Bool (strict)"("Visible"=w20) -> ()  [unwired: 2 in, 2 out]
      n475 = property on="21旅3" class="Bool (strict)"("Visible"=w20) -> ()  [unwired: 2 in, 2 out]
      n476 = property on="21旅4" class="Bool (strict)"("Visible"=w20) -> ()  [unwired: 2 in, 2 out]
      n477 = property on="22房1" class="Bool (strict)"("Visible"=w19) -> ()  [unwired: 2 in, 2 out]
      n478 = property on="22房2" class="Bool (strict)"("Visible"=w19) -> ()  [unwired: 2 in, 2 out]
      n479 = property on="22房3" class="Bool (strict)"("Visible"=w19) -> ()  [unwired: 2 in, 2 out]
      n480 = property on="22房4" class="Bool (strict)"("Visible"=w19) -> ()  [unwired: 2 in, 2 out]
      n481 = property on="22旅1" class="Bool (strict)"("Visible"=w19) -> ()  [unwired: 2 in, 2 out]
      n482 = property on="22旅2" class="Bool (strict)"("Visible"=w19) -> ()  [unwired: 2 in, 2 out]
      n483 = property on="22旅3" class="Bool (strict)"("Visible"=w19) -> ()  [unwired: 2 in, 2 out]
      n484 = property on="22旅4" class="Bool (strict)"("Visible"=w19) -> ()  [unwired: 2 in, 2 out]
      n485 = property on="23房1" class="Bool (strict)"("Visible"=w19) -> ()  [unwired: 2 in, 2 out]
      n486 = property on="23房2" class="Bool (strict)"("Visible"=w19) -> ()  [unwired: 2 in, 2 out]
      n487 = property on="23房3" class="Bool (strict)"("Visible"=w19) -> ()  [unwired: 2 in, 2 out]
      n488 = property on="23房4" class="Bool (strict)"("Visible"=w19) -> ()  [unwired: 2 in, 2 out]
      n489 = property on="23旅1" class="Bool (strict)"("Visible"=w19) -> ()  [unwired: 2 in, 2 out]
      n490 = property on="23旅2" class="Bool (strict)"("Visible"=w19) -> ()  [unwired: 2 in, 2 out]
      n491 = property on="23旅3" class="Bool (strict)"("Visible"=w19) -> ()  [unwired: 2 in, 2 out]
      n492 = property on="23旅4" class="Bool (strict)"("Visible"=w19) -> ()  [unwired: 2 in, 2 out]
      n493 = property on="25房1" class="Bool (strict)"("Visible"=w19) -> ()  [unwired: 2 in, 2 out]
      n494 = property on="25房2" class="Bool (strict)"("Visible"=w19) -> ()  [unwired: 2 in, 2 out]
      n495 = property on="25房3" class="Bool (strict)"("Visible"=w19) -> ()  [unwired: 2 in, 2 out]
      n496 = property on="25房4" class="Bool (strict)"("Visible"=w19) -> ()  [unwired: 2 in, 2 out]
      n497 = property on="25旅1" class="Bool (strict)"("Visible"=w19) -> ()  [unwired: 2 in, 2 out]
      n498 = property on="25旅2" class="Bool (strict)"("Visible"=w19) -> ()  [unwired: 2 in, 2 out]
      n499 = property on="25旅3" class="Bool (strict)"("Visible"=w19) -> ()  [unwired: 2 in, 2 out]
      n500 = property on="25旅4" class="Bool (strict)"("Visible"=w19) -> ()  [unwired: 2 in, 2 out]
      n501 = property on="26房1" class="Bool (strict)"("Visible"=w19) -> ()  [unwired: 2 in, 2 out]
      n502 = property on="26房2" class="Bool (strict)"("Visible"=w19) -> ()  [unwired: 2 in, 2 out]
      n503 = property on="26房3" class="Bool (strict)"("Visible"=w19) -> ()  [unwired: 2 in, 2 out]
      n504 = property on="26房4" class="Bool (strict)"("Visible"=w19) -> ()  [unwired: 2 in, 2 out]
      n505 = property on="26旅1" class="Bool (strict)"("Visible"=w19) -> ()  [unwired: 2 in, 2 out]
      n506 = property on="26旅2" class="Bool (strict)"("Visible"=w19) -> ()  [unwired: 2 in, 2 out]
      n507 = property on="26旅3" class="Bool (strict)"("Visible"=w19) -> ()  [unwired: 2 in, 2 out]
      n508 = property on="26旅4" class="Bool (strict)"("Visible"=w19) -> ()  [unwired: 2 in, 2 out]
      n509 = property on="27房1" class="Bool (strict)"("Visible"=w18) -> ()  [unwired: 2 in, 2 out]
      n510 = property on="27房2" class="Bool (strict)"("Visible"=w18) -> ()  [unwired: 2 in, 2 out]
      n511 = property on="27房3" class="Bool (strict)"("Visible"=w18) -> ()  [unwired: 2 in, 2 out]
      n512 = property on="27房4" class="Bool (strict)"("Visible"=w18) -> ()  [unwired: 2 in, 2 out]
      n513 = property on="27旅1" class="Bool (strict)"("Visible"=w18) -> ()  [unwired: 2 in, 2 out]
      n514 = property on="27旅2" class="Bool (strict)"("Visible"=w18) -> ()  [unwired: 2 in, 2 out]
      n515 = property on="27旅3" class="Bool (strict)"("Visible"=w18) -> ()  [unwired: 2 in, 2 out]
      n516 = property on="27旅4" class="Bool (strict)"("Visible"=w18) -> ()  [unwired: 2 in, 2 out]
      n517 = property on="29房1" class="Bool (strict)"("Visible"=w18) -> ()  [unwired: 2 in, 2 out]
      n518 = property on="29房2" class="Bool (strict)"("Visible"=w18) -> ()  [unwired: 2 in, 2 out]
      n519 = property on="29房3" class="Bool (strict)"("Visible"=w18) -> ()  [unwired: 2 in, 2 out]
      n520 = property on="29房4" class="Bool (strict)"("Visible"=w18) -> ()  [unwired: 2 in, 2 out]
      n521 = property on="29旅1" class="Bool (strict)"("Visible"=w18) -> ()  [unwired: 2 in, 2 out]
      n522 = property on="29旅2" class="Bool (strict)"("Visible"=w18) -> ()  [unwired: 2 in, 2 out]
      n523 = property on="29旅3" class="Bool (strict)"("Visible"=w18) -> ()  [unwired: 2 in, 2 out]
      n524 = property on="29旅4" class="Bool (strict)"("Visible"=w18) -> ()  [unwired: 2 in, 2 out]
